vi "Get Protocol Type.vi"(8 "error in (no error)":errorcluster, 11 "RS-xxx in":refnum<class "RS-xxx.lvclass">) -> (0 "error out":errorcluster, 2 "protocol type":T1=enum."AK RS-XXX", 3 "RS-xxx out":refnum<class "RS-xxx.lvclass">)   [LabVIEW 2018, in "Protocols.lvlib" / "RS-xxx.lvclass"]
doc: "Returns RS-XXX protocol type Enum.\n\nInput:\nRS-xxx in: represents an instance of the RS-xxx protocol class.\n\nOutput: \nRS-xxx out: represents an instance of the RS-xxx protocol class provided as input.\nProtocol Type: represents the type of the protocol in Enum format."
uses:
  RS-xxx.lvclass
  Protocol Parent/Types/Protocol Type.ctl
  Protocol Parent/Protocol Parent.lvclass
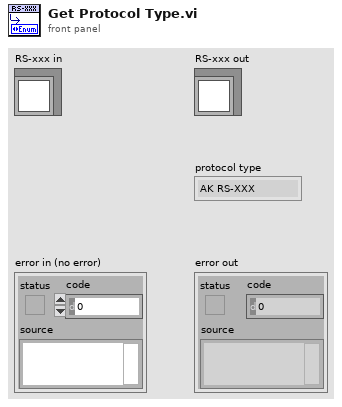
[diagram p1: front panel]
types:
  T1 = typedef "Protocols.lvlib/Protocol Parent.lvclass/Protocol Type.ctl" = enum16{"RS-XXX", "AK RS-XXX", "VISA", "TCPIP", "AK TCPIP", "UDP", "GPIB ConvBox"}
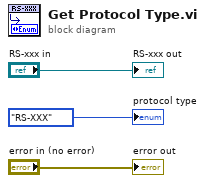
[diagram p0: block diagram]
diagram:
  "error out" <- "error in (no error)"
  "RS-xxx out" <- "RS-xxx in"
  "protocol type" <- Protocol_Type."RS-XXX" ("Protocol out")
